vi "Launch as Nested Panel.vi"(6 "timeout in ms (-1)":i32=-1, 8 "Error In":errorcluster, 9 "Panel":refnum<class "Panel.lvclass">, 10 "Panel To Launch":refnum<class "Panel Actor.lvclass">, 11 "Caller Actor in":refnum<class "Actor.lvclass">) -> (0 "Error Out":errorcluster, 2 "Actor's Enqueuer":refnum<class "Message Enqueuer.lvclass">, 3 "Caller Actor out":refnum<class "Actor.lvclass">)   [LabVIEW 2017, in "MGI-Panel Actor.lvlib"]
doc: "Launches a root panel as a nested actor of a non-panel actor.\n\n<B>Caller Actor In:</B> Nested caller Actor \n<B>Panel Actor In:</B> Panel actor to launch as nested actor\n<B>Panel:</B> Panel to use in displaying nested actor\n<B>timeout in ms</B> Time to wait for the panel to initialize\n<B>Error In:</B> Describes error conditions that occur before this node runs.\n\n<B>Caller Actor In:</B> Nested caller Actor \n<B>Actor's Enqueuer:</B> Enqueuer for newly spawned actor\n<B>Error Out:</B> Contains error information.\n----\nCopyright: MGI 2018\nAuthor: Derek Trepanier"
uses:
  MGI-Panel Actor.lvlib
  Panel Actor/Panel Actor.lvclass
  panel-manager/Source/Panel/Panel.lvclass
  <vilib>/ActorFramework/Actor/Actor.lvclass
  <vilib>/ActorFramework/Message Enqueuer/Message Enqueuer.lvclass
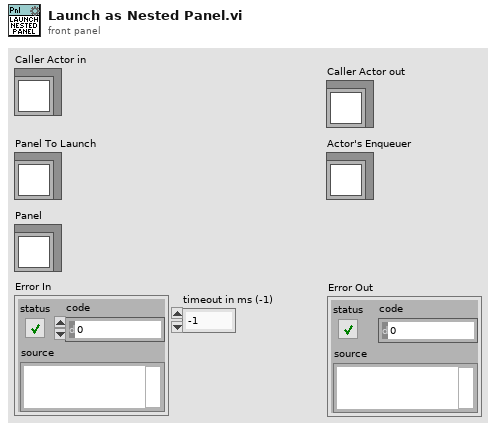
[diagram p1: front panel]
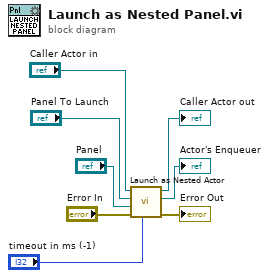
[diagram p0: block diagram]
diagram:
  n1 = call "Launch as Nested Actor.vi"("timeout in ms (-1)"="timeout in ms (-1)", "Error In"="Error In", "Panel"="Panel", "Panel Actor in"="Panel To Launch", "Caller Actor in"="Caller Actor in") -> ("Error Out"=→"Error Out":errorcluster, "Actor's Enqueuer"=→"Actor's Enqueuer":refnum<class "Message Enqueuer.lvclass">, "Caller Actor out"=→"Caller Actor out":refnum<class "Actor.lvclass">)  [unwired: 4 in]
